vi "Handle Error.vi"(8 "error in (no error)":errorcluster, 11 "UI Base in":refnum<class "UI Base.lvclass">) -> (0 "error out":errorcluster, 2 "stop actor?":bool=TRUE, 3 "UI Base out":refnum<class "UI Base.lvclass">)   [LabVIEW 2023, in "UI Base.lvlib" / "UI Base.lvclass"]
doc: "(<B>Filename</B>: Actor Framework.lvlib:Actor.lvclass:Handle Error.vi)\n\nDefines how the actor handles an error that occurred while processing a message. By default, this method does nothing except stop the actor."
uses:
  UI Base.lvclass
  UI Base.lvclass/UI Base.ctl
  <vilib>/ActorFramework/Actor/Actor.lvclass
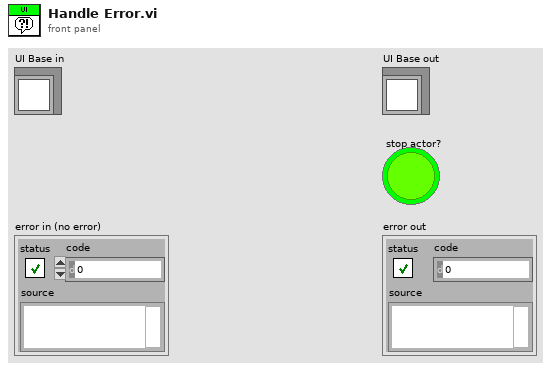
[diagram p1: front panel]
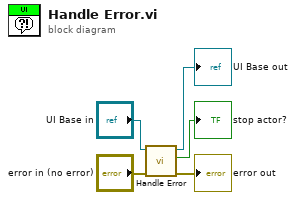
[diagram p0: block diagram]
diagram:
  n1 = call-parent "Handle Error.vi"("error in (no error)"="error in (no error)", "Actor in"="UI Base in") -> ("error out"=→"error out":errorcluster, "stop actor?"=→"stop actor?":bool, "Actor out"=→"UI Base out":refnum<class "UI Base.lvclass">)  [unwired: 7 in]
